vi "SRV_Hex String to Byte Array.vi"() -> ()   [LabVIEW 2014]
uses:
  SRV VIs/PacketMode/SRV_PM_Packet.ctl
panel:
  out "Extra Bytes":u8[](array[numeric]) format="%.0x"
  out "Packet Complete?":bool
  out "error out":errorcluster
  out "Packet Data dup":u8[](array[numeric]) format="%.0x"
  out "Packet":T1 {"Packet Data" format="%.0x"}
  out "size(s)":i32
  out "1D Array":u8[](array[numeric])=[255, 255, 254, 255, 255, 255] format="%.0x"
  in  "Hex string":string="FF FF FF FF 69 80 00 7D 6A 47 00 10 23 23 69 62 20 32 37 20 31 32 20 36 20 30 0D 0A C4 8B"
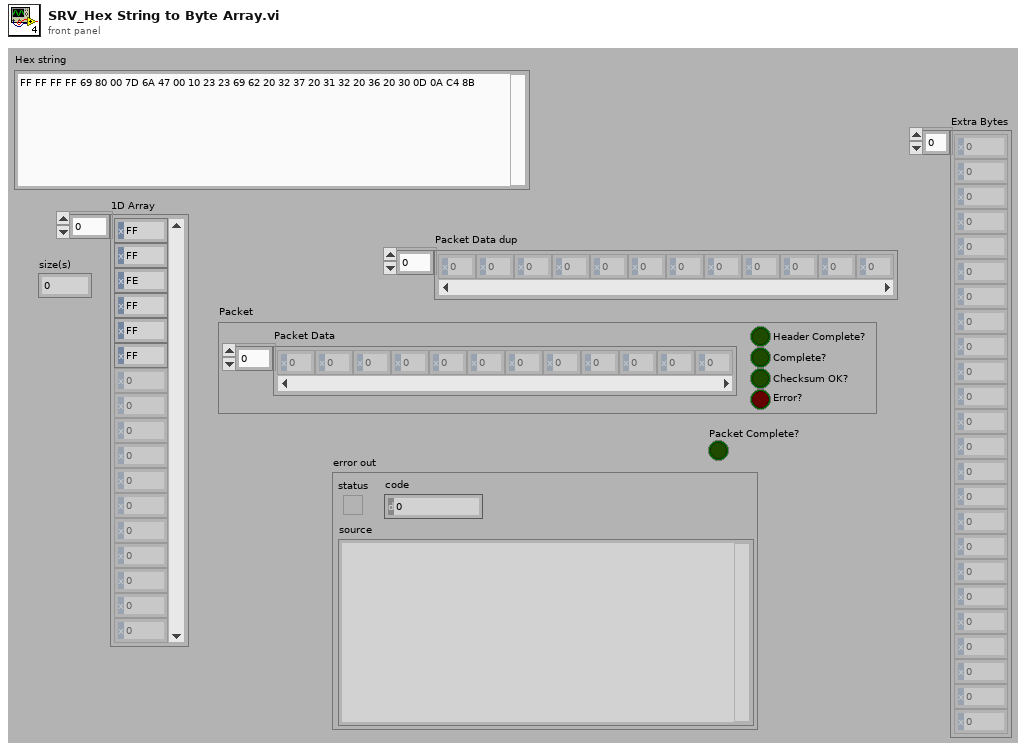
[diagram p1: front panel]
types:
  T1 = typedef "SRV_PM_Packet.ctl" = cluster{"Packet Data":u8[], "Header Complete?":bool, "Complete?":bool, "Checksum OK?":bool, "Error?":bool}
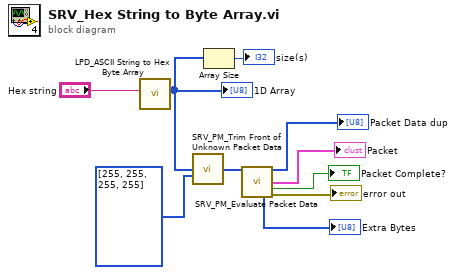
[diagram p0: block diagram]
diagram:
  n1 = call "LPD_ASCII String to Hex Byte Array.vi"("String"="Hex string") -> ("Hex Byte Array"=w7:u8[])  [unwired: 10 in]
  "1D Array" <- w7
  n2 = call "SRV_PM_Trim Front of Unknown Packet Data.vi"("1D Array"=w7, "Search"=u8[] [255, 255, 255, 255]) -> ("Trimmed 1D Array"=w6:u8[])  [unwired: 12 in, 1 out]
  n3 = Array Size(array=w7) -> (size(s)=→"size(s)":i32)
  n4 = call "SRV_PM_Evaluate Packet Data.vi"("Packet Data"=w6) -> ("Packet Data dup"=→"Packet Data dup":u8[], "Packet"=→"Packet":T1, "Packet Complete?"=→"Packet Complete?":bool, "Extra Bytes"=→"Extra Bytes":u8[], "error out"=→"error out":errorcluster)  [unwired: 10 in]
